vi "Create Panel by Type.vi"(5 "Display Class Type":refnum<class "Panel.lvclass">, 7 "Panel Type":refnum<class "Panel.lvclass">, 8 "error in (no error)":errorcluster, 9 "Run? (T)":bool=TRUE, 11 "Manager in":refnum<class "Manager.lvclass">) -> (0 "error out":errorcluster, 2 "Panel":refnum<class "Panel.lvclass">, 3 "Manager out":refnum<class "Manager.lvclass">)   [LabVIEW 2014, in "OOPanel.lvlib" / "Manager.lvclass"]
uses:
  Manager.lvclass
  Panel/Panel.lvclass
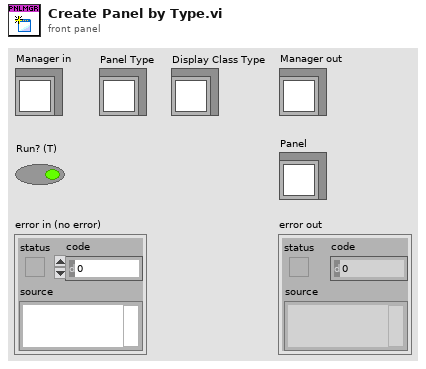
[diagram p1: front panel]
types:
  T1 = typedef "OOPanel.lvlib/Manager.lvclass/Ref Data.ctl" = cluster{"SubPanel Map":T2, "Panels":refnum<class "Panel.lvclass">[]}
  T2 = typedef "OOPanel.lvlib/Manager.lvclass/SubPanel Map.ctl" = cluster{"SubPanels":refnum<vi>[], "Panels":refnum<class "Panel.lvclass">[]}
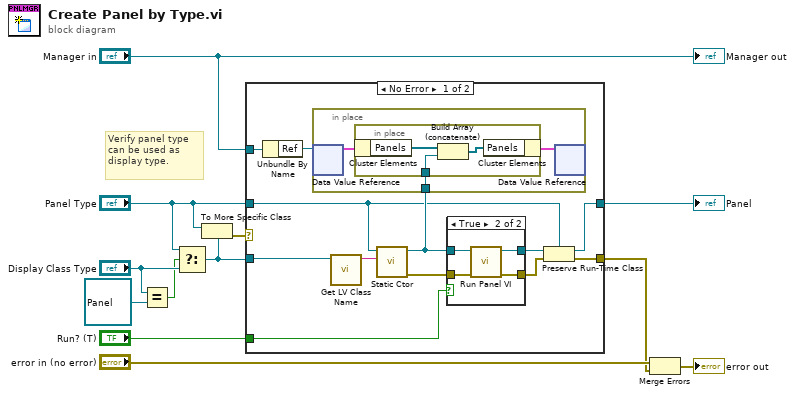
[diagram p0: block diagram]
diagram:
  # "Verify panel type can be used as display type."
  n1 = Equal?(x="Display Class Type", y=refnum<class "Panel.lvclass"> refnum ("Display Class Type")) -> (x = y?=w4:bool)
  n2 = Select(t="Panel Type", s=w4, f="Display Class Type") -> (s? t:f=w2:refnum<class "Panel.lvclass">)
  n3 = To More Specific Class(target class=w2, reference="Panel Type") -> (error out=w1:errorcluster)  [unwired: 1 in, 1 out]
  n4 = case shown="No Error" w1 {
    selector: w1 -> [_ w37]
    tunnel: "Manager in" -> [w23 _]
    tunnel: [w22 w38] -> w11
    tunnel: "Run? (T)" -> [w17 _]
    tunnel: [w16 w37] -> w8
    tunnel: "Panel Type" -> [w14 w38]
    tunnel: w2 -> [w13 _]
    frame No Error {
      n5 = Unbundle By Name(w23) -> ("Ref"=w24:refnum<data-value>)
      n6 = call <vilib>:"Get LV Class Name.vi"("object"=w13) -> ("class name"=w15:string)  [unwired: 9 in, 1 out]
      n7 = call "Static Ctor.vi"("Display-As"=w15, "Panel in"=w14) -> ("error out"=w21:errorcluster, "Panel out"=w20:refnum<class "Panel.lvclass">)  [unwired: 8 in]
      n8 = in-place {
        in-place-border: w20 -> [w25]
        n9 = in-place-dvr #1(w24) -> (w27:T1)  [unwired: 1 out]
        n10 = in-place {
          in-place-border: w25 -> [w29]
          n11 = in-place-cluster #2(w27) -> ("Panels"=w30:refnum<class "Panel.lvclass">[])
          n12 = Build Array (concatenate)(w30, w29) -> (w28:refnum<class "Panel.lvclass">[])
          n13 = in-place-cluster #2("Panels"=w28) -> (w26:T1)
        }
        n14 = in-place-dvr #1(w26) -> ()  [unwired: 2 out]
      }
      n15 = case shown="True" w17 {
        tunnel: w21 -> [w31 w36]
        tunnel: w20 -> [w32 w35]
        tunnel: [w32 w34] -> w19
        tunnel: [w31 w33] -> w18
        frame False {
        }
        frame True {
          n16 = call "Run Panel VI.vi"("error in (no error)"=w36, "Panel in"=w35) -> ("error out"=w33:errorcluster, "Panel out"=w34:refnum<class "Panel.lvclass">)  [unwired: 8 in]
        }
      }
      n17 = Preserve Run-Time Class(object in=w19, error in=w18, 2:w14) -> (object out=w22:refnum<class "Panel.lvclass">, error out=w16:errorcluster)
    }
    frame Error {
    }
  }
  "Panel" <- w11
  n18 = Merge Errors("error in (no error)", w8) -> (→"error out":errorcluster)
  "Manager out" <- "Manager in"
